vi "SCOPE_GetSettings.vi"(8 "error in (no error)":errorcluster, 10 "Configuration Cluster":T1={"General"={"Config.ini"=path "", "Default Logging Path"=path ""}, "Hardware"={"Global T VAR"="", "Global B VAR"="", "VISAS"={"GEN COM"="", "SCOPE COM"="", "VNA COM"=""}, "Connected?"={"SCOPE"=FALSE, "GEN"=FALSE, "VNA"=FALSE}}, "Operation"={"Operation Mode"=enum."Idle-Off", "Status"="", "NewLog?"=FALSE, "OvenWarn"=FALSE, "Scope Settings"={"TimeBase"=0.0, "VerticalScale"=4.0, "Channel"=enum."Channel 2"}, "Gen Settings"={"Amplitude"=0.0, "Frequency"=0.0, "Offset"=0.0}}}) -> (0 "error out":errorcluster, 2 "Configuration Cluster Out":T1={"General"={"Config.ini"=path "", "Default Logging Path"=path ""}, "Hardware"={"Global T VAR"="", "Global B VAR"="", "VISAS"={"GEN COM"="", "SCOPE COM"="", "VNA COM"=""}, "Connected?"={"SCOPE"=FALSE, "GEN"=FALSE, "VNA"=FALSE}}, "Operation"={"Operation Mode"=enum."Idle-Off", "Status"="", "NewLog?"=FALSE, "OvenWarn"=FALSE, "Scope Settings"={"TimeBase"=0.0, "VerticalScale"=4.0, "Channel"=enum."Channel 2"}, "Gen Settings"={"Amplitude"=0.0, "Frequency"=0.0, "Offset"=0.0}}})   [LabVIEW 2021]
uses:
  Config_Cluster.ctl
  Mode_Enum.ctl
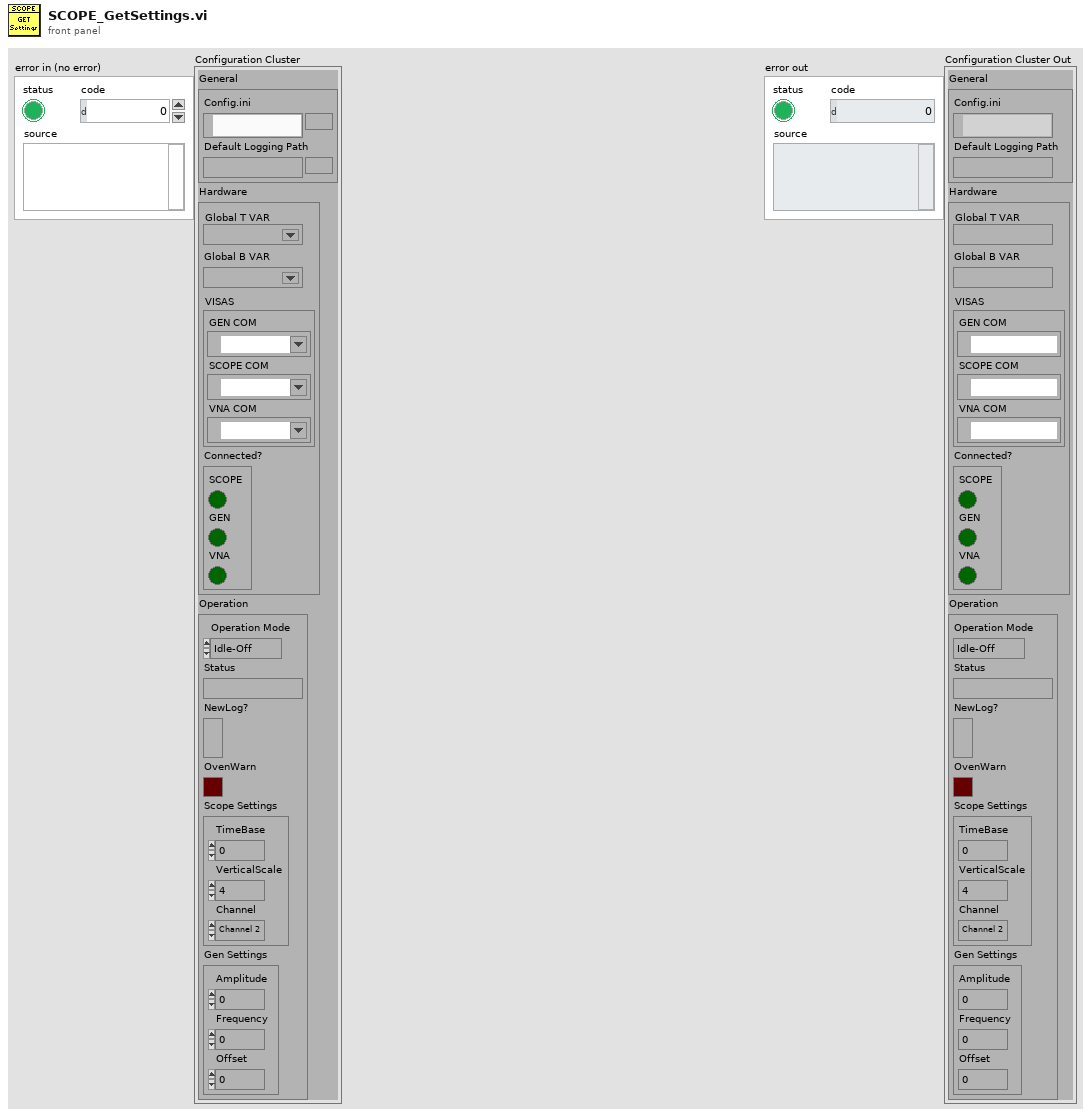
[diagram p1: front panel]
types:
  T1 = typedef "Config_Cluster.ctl" = cluster{"General":cluster{"Config.ini":path, "Default Logging Path":path}, "Hardware":cluster{"Global T VAR":refnum<k21>, "Global B VAR":refnum<k21>, "VISAS":cluster{"GEN COM":refnum<visa-resource-name>, "SCOPE COM":refnum<visa-resource-name>, "VNA COM":refnum<visa-resource-name>}, "Connected?":cluster{"SCOPE":bool, "GEN":bool, "VNA":bool}}, "Operation":cluster{"Operation Mode":T2, "Status":string, "NewLog?":bool, "OvenWarn":bool, "Scope Settings":cluster{"TimeBase":dbl, "VerticalScale":dbl, "Channel":enum16{"Channel 2", "Channel 1"}}, "Gen Settings":cluster{"Amplitude":dbl, "Frequency":dbl, "Offset":dbl}}}
  T2 = typedef "Mode_Enum.ctl" = enum16{"Logging", "Idle-Off", "Idle"}
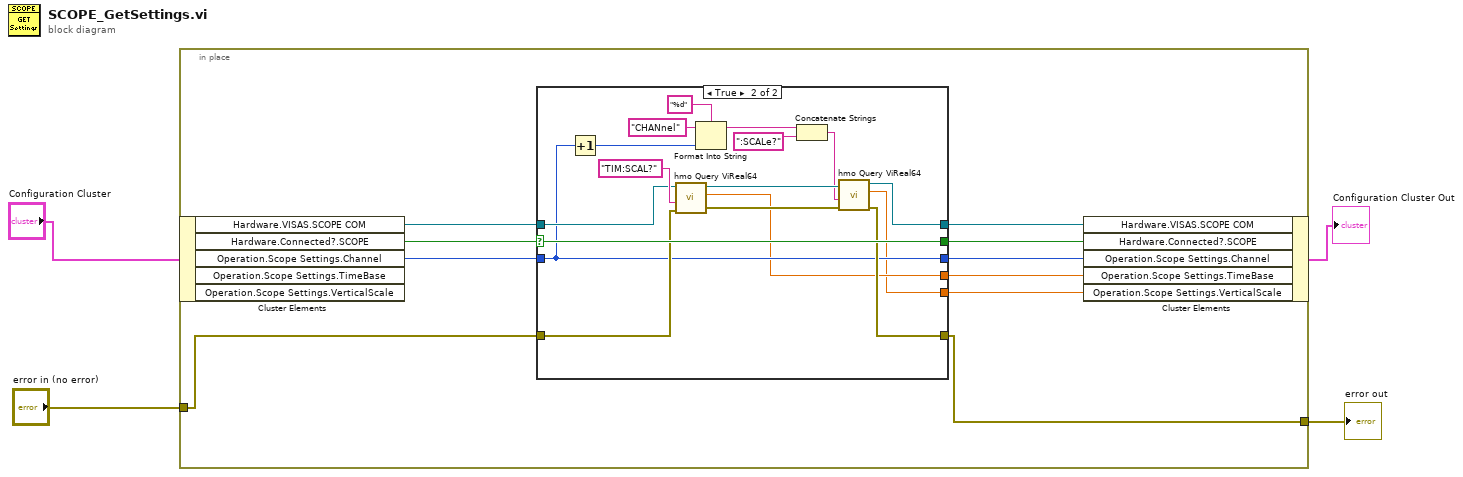
[diagram p0: block diagram]
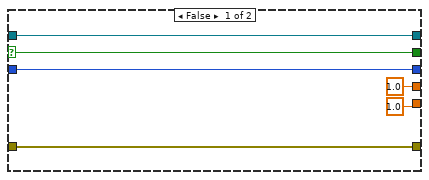
[diagram p2: hidden frame]
diagram:
  n1 = in-place {
    in-place-border: "error in (no error)" -> [w11]
    in-place-border: [w10] -> w1
    n2 = in-place-cluster #1("Configuration Cluster") -> ("Hardware.VISAS.SCOPE COM"=w13:refnum<visa-resource-name>, "Hardware.Connected?.SCOPE"=w14:bool, "Operation.Scope Settings.Channel"=w8:enum16{"Channel 2", "Channel 1"})  [unwired: 2 out]
    n3 = case shown="True" w14 {
      selector: w14 -> [w20 w37]
      tunnel: w13 -> [w18 w33]
      tunnel: [w20 w37] -> w12
      tunnel: w11 -> [w19 w30]
      tunnel: [w19 w31] -> w10
      tunnel: [w18 w32] -> w9
      tunnel: w8 -> [w15 w26]
      tunnel: [w15 w26] -> w7
      tunnel: [1.0 ("Response Value") w22] -> w6
      tunnel: [1.0 ("Response Value") w21] -> w5
      frame False {
      }
      frame True {
        n4 = Increment(x=w26) -> (x+1=w27:enum16{"Channel 2", "Channel 1"})
        n5 = call <instrlib>:"hmo Query ViReal64.vi"("error in (no error)"=w30, "Query"="TIM:SCAL?", "VISA resource name"=w33) -> ("error out"=w36:errorcluster, "Response Value"=w22:dbl, "VISA resource name out"=w35:refnum<visa-resource-name>)  [unwired: 6 in]
        n6 = Format Into String(format string="%d", initial string="CHANnel", w27) -> (resulting string=w28:string)  [unwired: 1 in, 1 out]
        n7 = Concatenate Strings(w28, ":SCALe?" ("string")) -> (w23:string)
        n8 = call <instrlib>:"hmo Query ViReal64.vi"("error in (no error)"=w36, "Query"=w23, "VISA resource name"=w35) -> ("error out"=w31:errorcluster, "Response Value"=w21:dbl, "VISA resource name out"=w32:refnum<visa-resource-name>)  [unwired: 6 in]
      }
    }
    n9 = in-place-cluster #1("Hardware.VISAS.SCOPE COM"=w9, "Hardware.Connected?.SCOPE"=w12, "Operation.Scope Settings.Channel"=w7, "Operation.Scope Settings.TimeBase"=w6, "Operation.Scope Settings.VerticalScale"=w5) -> (→"Configuration Cluster Out":T1)
  }
  "error out" <- w1
